vi "Get Consumer Values.vi"(8 "error in":errorcluster, 11 "Device Cluster.lvclass in":refnum<class "Device Cluster.lvclass">) -> (0 "error out":errorcluster, 1 "Consumer Ch":T2[](array[typedef]), 2 "Consumer Control":T1, 3 "Device Cluster.lvclass out":refnum<class "Device Cluster.lvclass">)   [LabVIEW 2023, in "Device Cluster.lvclass"]
uses:
  Device Cluster.lvclass
  Consumer Ch.ctl
  Consumer Control.ctl
  Device Cluster.lvclass/Device Cluster.ctl
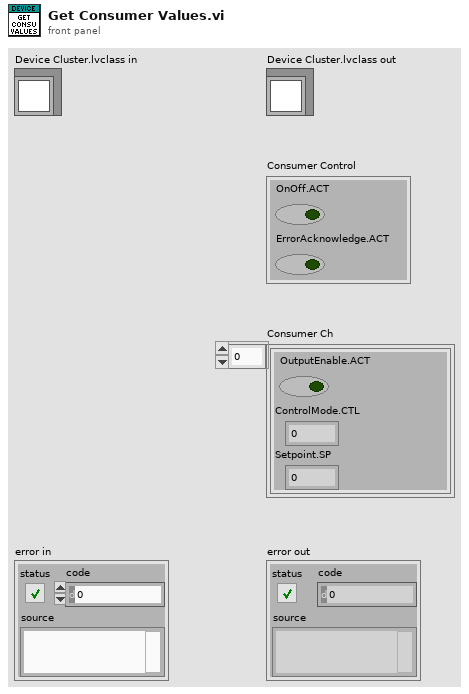
[diagram p1: front panel]
types:
  T1 = typedef "Device Cluster.lvclass/Consumer Control.ctl" = cluster{"OnOff.ACT":bool, "ErrorAcknowledge.ACT":bool}
  T2 = typedef "Device Cluster.lvclass/Consumer Ch.ctl" = cluster{"OutputEnable.ACT":bool, "ControlMode.CTL":u16, "Setpoint.SP":dbl}
  T3 = typedef "Cluster.lvclass/Consumer Control.ctl" = cluster{"OnOff.ACT":bool, "ErrorAcknowledge.ACT":bool}
  T4 = typedef "Cluster.lvclass/Consumer Ch.ctl" = cluster{"OutputEnable.ACT":bool, "ControlMode.CTL":u16, "Setpoint.SP":dbl}
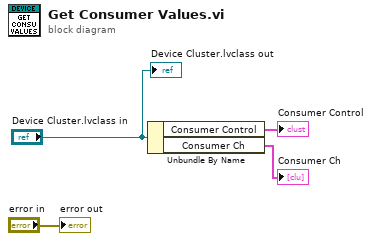
[diagram p0: block diagram]
diagram:
  n1 = Unbundle By Name("Device Cluster.lvclass in") -> ("Consumer Control"=→"Consumer Control":T3, "Consumer Ch"=→"Consumer Ch":T4[])
  "Device Cluster.lvclass out" <- "Device Cluster.lvclass in"
  "error out" <- "error in"
